vi "Get path from registry.vi"(9 "Name":string, 10 "Type":string, 11 "Registry":T1) -> (2 "Found?":bool, 3 "Path":string)   [LabVIEW 2014]
uses:
  Registry.ctl
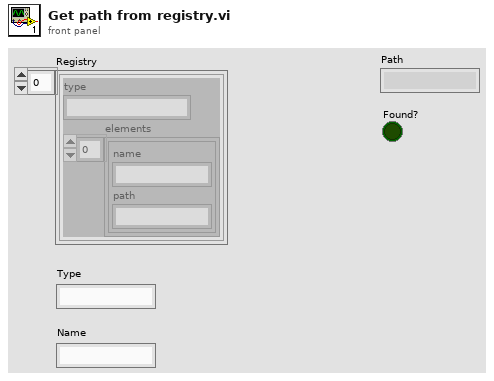
[diagram p1: front panel]
types:
  T1 = typedef "Registry.ctl" = cluster{"type":string, "elements":cluster{"name":string, "path":string}[]}[]
  T2 = cluster{"type":string, "elements":cluster{"name":string, "path":string}[]}
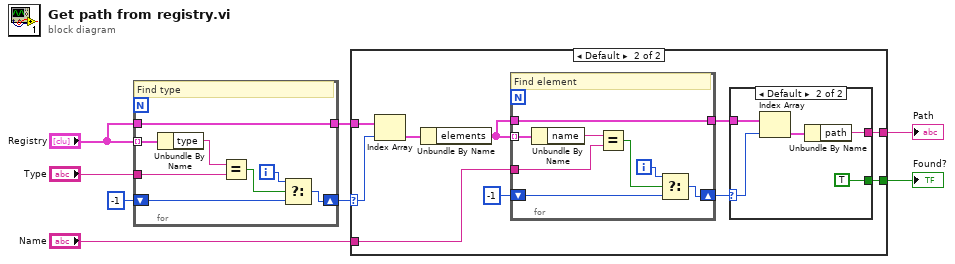
[diagram p0: block diagram]
diagram:
  n1 = for {
    tunnel: "Registry" -> [w16] mode=indexing
    tunnel: "Type" -> [w14]
    shift-right: [w12] -> w5
    shift-left: -1 -> [w10]
    tunnel: [w9] -> w3
    tunnel: "Registry" -> [w9]
    i -> [w11]
    # "Find type"
    n2 = Unbundle By Name(w16) -> ("type"=w15:string)
    n3 = Equal?(x=w15, y=w14) -> (x = y?=w13:bool)
    n4 = Select(t=w11, s=w13, f=w10) -> (s? t:f=w12:i32)
  }
  n5 = case shown="Default" w5 {
    selector: w5 -> [_ w23]
    tunnel: "Name" -> [_ w26]
    tunnel: w3 -> [_ w21]
    tunnel: [_ w18] -> w2
    tunnel: [_ w17] -> w1
    frame -1 {
    }
    frame Default {
      n6 = Index Array(array=w21, index=w23) -> (element=w24:T2)
      n7 = Unbundle By Name(w24) -> ("elements"=w20:cluster{"name":string, "path":string}[])
      n8 = for {
        tunnel: w20 -> [w39] mode=indexing
        tunnel: w26 -> [w37]
        shift-right: [w35] -> w22
        shift-left: -1 ("y") -> [w33]
        tunnel: [w32] -> w19
        tunnel: w20 -> [w32]
        i -> [w34]
        # "Find element"
        n9 = Unbundle By Name(w39) -> ("name"=w38:string)
        n10 = Equal?(x=w38, y=w37) -> (x = y?=w36:bool)
        n11 = Select(t=w34, s=w36, f=w33) -> (s? t:f=w35:i32)
      }
      n12 = case shown="Default" w22 {
        selector: w22 -> [_ w30]
        tunnel: w19 -> [_ w31]
        tunnel: [_ w28] -> w18
        tunnel: [_ TRUE] -> w17
        frame -1 {
        }
        frame Default {
          n13 = Index Array(array=w31, index=w30) -> (element=w29:cluster{"name":string, "path":string})
          n14 = Unbundle By Name(w29) -> ("path"=w28:string)
        }
      }
    }
  }
  "Path" <- w2
  "Found?" <- w1
